vi "Options Parser Example.vi"() -> ()   [LabVIEW 2011]
doc: "VI to interactive try out the options parser as part of G CLI."
uses:
  Argument Parser/Option Class/Option Configuration.ctl
  Argument Parser/Option Class/Argument Type.ctl
  Argument Parser/Option Set Class/Option Set.lvclass
  Argument Parser/Option Class/Option.lvclass
panel:
  out "Option2 Value":string
  out "Option2 Set":bool
  out "Option1 Value":string
  out "Option1 Set":bool
  out "Trailing Arguments":string[](array[string])
  in  "Arguments":string[](array[string])=["-o", "Value", "File.txt", "File2.txt"]
  in  "Options":T1[](array[typedef])=[{"Option Type"=enum."value", "Option Labels"=["o"], "Key"="Option1", "Description"="Example Option", "Required"=FALSE, "Default Value"="Default"}, {"Option Type"=enum."flag", "Option Labels"=["o2", "opt2"], "Key"="Option2", "Description"="Another Example", "Required"=FALSE, "Default Value"=""}]
  # "Outputs"
  # "Inputs"
  # "Instructions"
  # "1. Setup the options you expect or leave as default. This sets up 2 options called option 1 (-o)\n    and Option2 (-o2 or -opt2). Option 2 is a flag so has no value field.\n2. In the arguments array at the top put in the input arguments. to set option1 put -o in one\n    and the value in the next. To set Option2 just include a -o2.\n3. Run the VI and see the outputs update. Option1 and Option2 will show if they are set and\n    what the value is. Any additioanl arguments are shown belo."
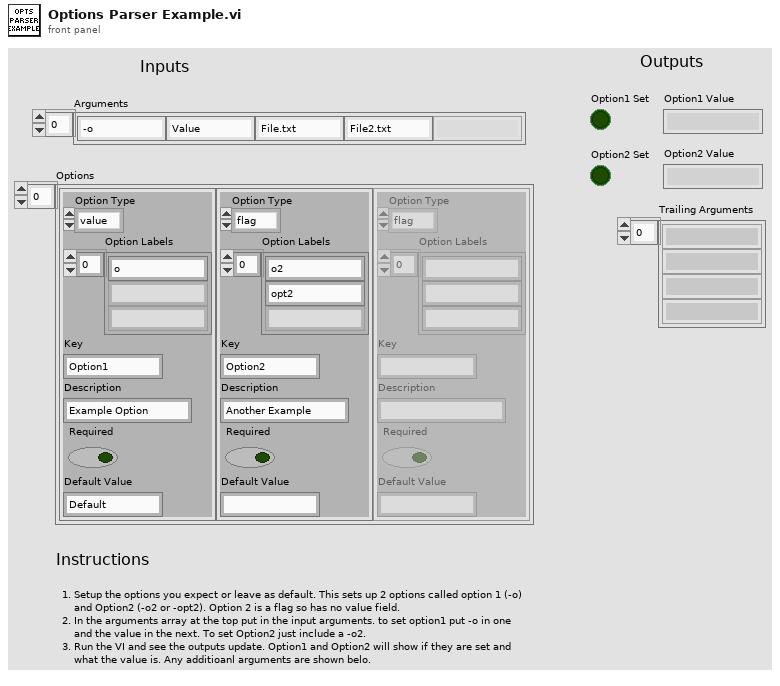
[diagram p1: front panel]
types:
  T1 = typedef "Option Parser.lvlib/Option.lvclass/Option Configuration.ctl" = cluster{"Option Type":T2, "Option Labels":string[], "Key":string, "Description":string, "Required":bool, "Default Value":string}
  T2 = typedef "Option Parser.lvlib/Option.lvclass/Argument Type.ctl" = enum16{"flag", "value"}
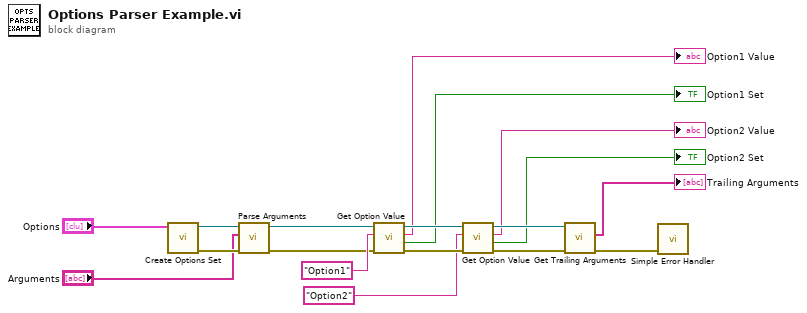
[diagram p0: block diagram]
diagram:
  n1 = call "Create Options Set.vi"("Options"="Options") -> ("error out"=w15:errorcluster, "Option Set out"=w16:refnum<class "Option Set.lvclass">)  [unwired: 9 in]
  n2 = call "Parse Arguments.vi"("error in (no error)"=w15, "Arguments"="Arguments", "Option Set in"=w16) -> ("error out"=w12:errorcluster, "Option Set out"=w13:refnum<class "Option Set.lvclass">)  [unwired: 5 in, 2 out]
  n3 = call "Get Option Value.vi"("error in (no error)"=w12, "Option Key"="Option1", "Option Set in"=w13) -> ("error out"=w11:errorcluster, "Set"=→"Option1 Set":bool, "Value"=→"Option1 Value":string, "Option Set out"=w7:refnum<class "Option Set.lvclass">)  [unwired: 5 in]
  n4 = call "Get Option Value.vi"("error in (no error)"=w11, "Option Key"="Option2", "Option Set in"=w7) -> ("error out"=w8:errorcluster, "Set"=→"Option2 Set":bool, "Value"=→"Option2 Value":string, "Option Set out"=w6:refnum<class "Option Set.lvclass">)  [unwired: 5 in]
  n5 = call "Get Trailing Arguments.vi"("error in (no error)"=w8, "Option Set in"=w6) -> ("error out"=w10:errorcluster, "Arguments"=→"Trailing Arguments":string[])  [unwired: 7 in, 1 out]
  n6 = call <vilib>:"Simple Error Handler.vi"("error in (no error)"=w10) -> ()  [unwired: 4 in, 5 out]
